vi "Validate Fixed Header.vi"(11 "Fixed Header":u8 format="%08b") -> (1 "Valid":bool, 2 "Control Packet Type":T1, 3 "Fixed Header dup":u8 format="%08b")   [LabVIEW 2013]
uses:
  Control Packet Type -- enum.ctl
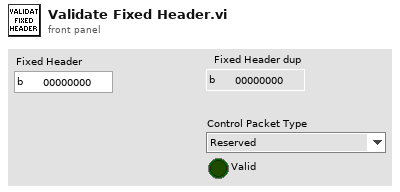
[diagram p1: front panel]
types:
  T1 = typedef "Control Packet Type -- enum.ctl" = enum16{"Reserved", "CONNECT", "CONNACK", "PUBLISH", "PUBACK", "PUBREC", "PUBREL", "PUBCOMP", "SUBSCRIBE", "SUBACK", "UNSUBSCRIBE", "UNSUBACK", "PINGREQ", "PINGRESP", "DISCONNECT", "Reserved(15)"}
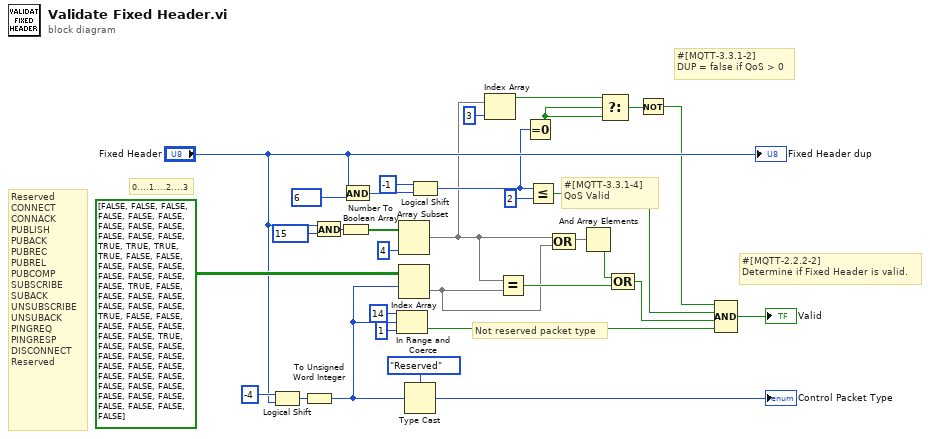
[diagram p0: block diagram]
diagram:
  # "Not reserved packet type"
  # "#[MQTT-3.3.1-2]\nDUP = false if QoS > 0"
  # "#[MQTT-3.3.1-4]\nQoS Valid"
  # "#[MQTT-2.2.2-2]\nDetermine if Fixed Header is valid."
  # "0....1....2....3"
  # "Reserved\nCONNECT\nCONNACK\nPUBLISH\nPUBACK\nPUBREC\nPUBREL\nPUBCOMP\nSUBSCRIBE\nSUBACK\nUNSUBSCRIBE\nUNSUBACK\nPINGREQ\nPINGRESP\nDISCONNECT\nReserved"
  n1 = Logical Shift(y=i16 -4, x="Fixed Header") -> (x << y=w25:u8)
  n2 = To Unsigned Word Integer(number=w25) -> (unsigned 16bit integer=w21:u16)
  n3 = And(x="Fixed Header", y=u8 15) -> (x .and. y?=w31:u8)
  n4 = Number To Boolean Array(number=w31) -> (Boolean array=w15:bool[])
  n5 = And(x="Fixed Header", y=u8 6) -> (x .and. y?=w11:u8)
  n6 = In Range and Coerce(upper limit=u16 14, x=w21, lower limit=u16 1) -> (In Range?=w24:bool)  [unwired: 1 out]
  n7 = Array Subset(array=w15, length=4) -> (w6:bool[])  [unwired: 1 in]
  n8 = Index Array(array=bool[][] [[FALSE, FALSE, FALSE, FALSE], [FALSE, FALSE, FALSE, FALSE], [FALSE, FALSE, FALSE, FALSE], [TRUE, TRUE, TRUE, TRUE], [FALSE, FALSE, FALSE, FALSE], [FALSE, FALSE, FALSE, FALSE], [FALSE, TRUE, FALSE, FALSE], [FALSE, FALSE, FALSE, FALSE], [FALSE, TRUE, FALSE, FALSE], [FALSE, FALSE, FALSE, FALSE], [FALSE, TRUE, FALSE, FALSE], [FALSE, FALSE, FALSE, FALSE], [FALSE, FALSE, FALSE, FALSE], [FALSE, FALSE, FALSE, FALSE], [FALSE, FALSE, FALSE, FALSE], [FALSE, FALSE, FALSE, FALSE]] ("Boolean array"), index (row)=w21) -> (element=w14:bool[])  [unwired: 1 in]
  n9 = Type Cast(type=Control_Packet_Type_--_enum."Reserved" ("Control Packet Type"), x=w21) -> (*(type *) &x=→"Control Packet Type":T1)
  n10 = Logical Shift(y=i16 -1, x=w11) -> (x << y=w7:u8)
  n11 = Index Array(array=w6, index=3) -> (element=w4:bool)
  n12 = Equal?(x=w6, y=w14) -> (x = y?=w19:bool)
  n13 = Equal To 0?(x=w7) -> (x = 0?=w3:bool)
  n14 = Less Or Equal?(x=w7, y=u8 2) -> (x <= y?=w8:bool)
  n15 = Compound Arithmetic op=OR(w6, w14) -> (w20:bool[])
  n16 = And Array Elements(Boolean array=w20) -> (logical AND=w18:bool)
  n17 = Select(t=w4, s=w3, f=w3) -> (s? t:f=w2:bool)
  n18 = Compound Arithmetic op=OR(w18, w19) -> (w17:bool)
  n19 = Not(x=w2) -> (.not. x?=w1:bool)
  n20 = Compound Arithmetic op=AND(w1, w8, w17, w24) -> (→"Valid":bool)
  "Fixed Header dup" <- "Fixed Header"
